vi "1_1_2.vi"() -> ()   [LabVIEW 2023, in "2025.lvlib"]
uses:
  2025.lvlib
panel:
  out "counter":i32
  out "Gauge":i32(knob)=16 scale=0.0..99.0
  out "Numeric 3":i32
  out "index of element":i32
  out "min index(es)":i32
  out "min value":i32
  out "max index(es)":i32
  out "max value":i32
  out "String":string
  out "iteration":i32
  out "Numeric 2":i32
  out "RIGHT = ON":bool
  out "x+y":i32
  out "x-y*floor(x/y)":i32
  out "floor(x/y)":i32
  out "Numeric":i32
  in  "s":bool
  out "size(s)":i32
  out "Array":i32[](array[numeric])
  # "2666 too low"
  # "6707 too high"
  # "6248 too low"
  # "6266 not it"
  # "6706 TOO HIGH"
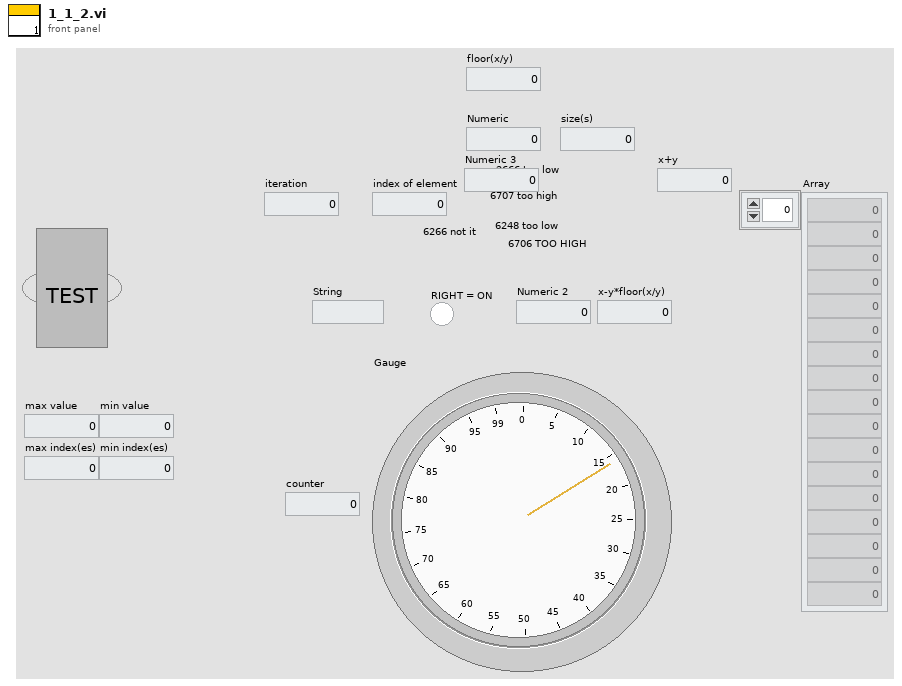
[diagram p1: front panel]
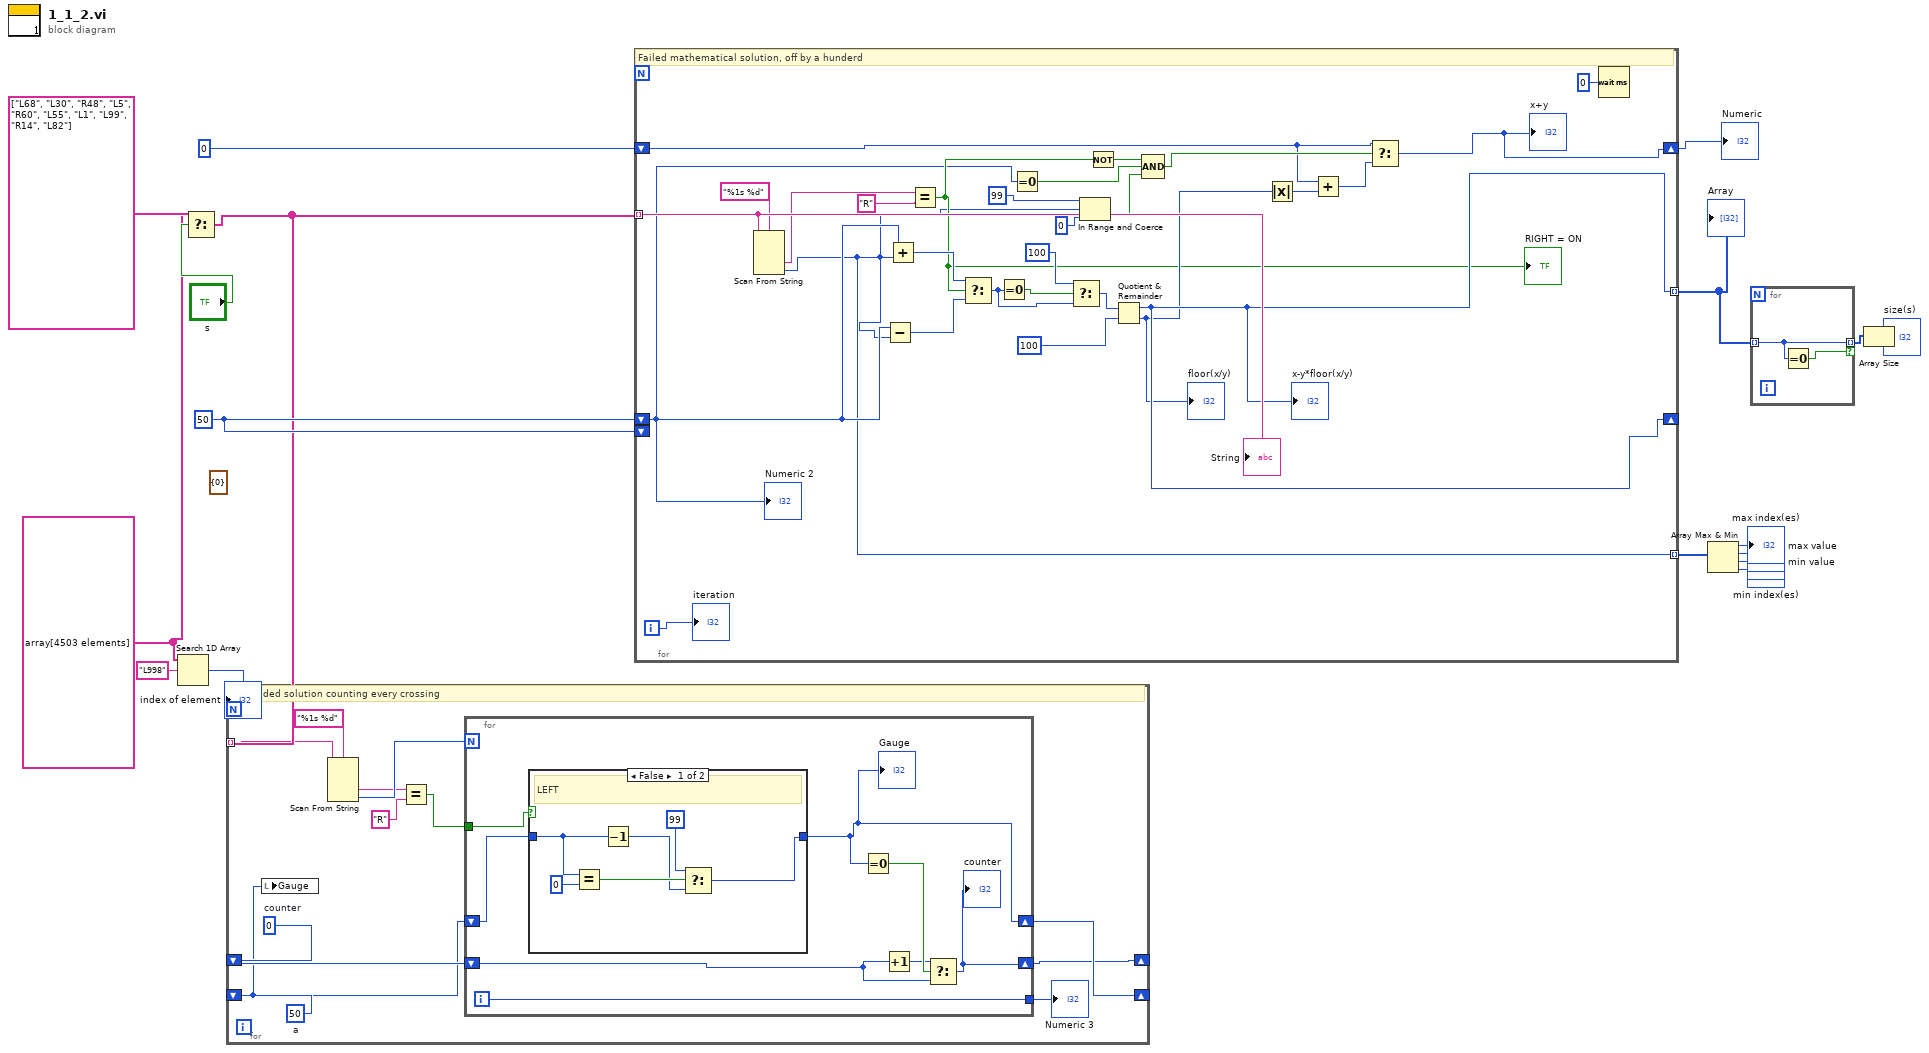
[diagram p0: block diagram]
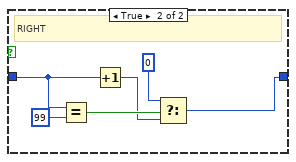
[diagram p2: hidden frame]
diagram:
  w1 = 0  # counter
  w2 = 50  # a
  (unwired) cluster{"b":i32} {"b"=0} ("Gauge")
  w6 = string[] array[4503 elements]
  w12 = 50
  n1 = Search 1D Array(1D array=w6, element="L998") -> (index of element=→"index of element":i32)  [unwired: 1 in]
  n2 = Select(t=w6, s="s", f=string[] ["L68", "L30", "R48", "L5", "R60", "L55", "L1", "L99", "R14", "L82"]) -> (s? t:f=w3:string[])
  n3 = for {
    tunnel: w3 -> [w29] mode=indexing
    shift-right: [w23] -> _
    shift-left: w2 -> [w20]
    shift-right: [w21] -> _
    shift-left: w1 -> [w22]
    # "hardcoded solution counting every crossing"
    n4 = local write "Gauge"(w20) -> ()
    n5 = Scan From String(format string="%1s %d", input string=w29) -> (output 1=w26:string, output 2=w28:i32)  [unwired: 4 in, 3 out]
    n6 = Equal?(x=w26, y="R") -> (x = y?=w25:bool)
    n7 = for {
      N: w28 -> [_]
      tunnel: [w38] -> w27
      tunnel: w25 -> [w37]
      shift-right: [w31] -> w23
      shift-left: w20 -> [w36]
      shift-right: [w35] -> w21
      shift-left: w22 -> [w33]
      i -> [w38]
      n8 = case shown="False" w37 {
        tunnel: w36 -> [w44 w50]
        tunnel: [w40 w46] -> w31
        frame False {
          # "LEFT"
          n9 = Equal?(x=w44, y=0) -> (x = y?=w42:bool)
          n10 = Decrement(x=w44) -> (x-1=w41:i32)
          n11 = Select(t=99, s=w42, f=w41) -> (s? t:f=w40:i32)
        }
        frame True {
          # "RIGHT"
          n12 = Equal?(x=w50, y=99) -> (x = y?=w48:bool)
          n13 = Increment(x=w50) -> (x+1=w47:i32)
          n14 = Select(t=0 ("y"), s=w48, f=w47) -> (s? t:f=w46:i32)
        }
      }
      "Gauge" <- w31
      n15 = Equal To 0?(x=w31) -> (x = 0?=w34:bool)
      n16 = Increment(x=w33) -> (x+1=w32:i32)
      n17 = Select(t=w32, s=w34, f=w33) -> (s? t:f=w35:i32)
      "counter" <- w35
    }
    "Numeric 3" <- w27
  }
  n18 = for {
    tunnel: w3 -> [w78] mode=indexing
    shift-right: [w68] -> _
    shift-left: w12 -> [w60]
    tunnel: [w68] -> w13 mode=indexing
    shift-right: [w52] -> w14
    shift-left: 0 -> [w54]
    shift-left: w12 -> [_]
    tunnel: [w51] -> w11 mode=indexing
    i -> [w69]
    # "Failed mathematical solution, off by a hunderd"
    n19 = Scan From String(format string="%1s %d", input string=w78) -> (output 1=w76:string, output 2=w51:i32)  [unwired: 4 in, 3 out]
    n20 = Subtract(x=w60, y=w51) -> (x-y=w73:i32)
    n21 = Add(x=w60, y=w51) -> (x+y=w74:i32)
    n22 = Equal?(x=w76, y="R") -> (x = y?=w62:bool)
    "RIGHT = ON" <- w62
    n23 = Select(t=w74, s=w62, f=w73) -> (s? t:f=w63:i32)
    n24 = Equal To 0?(x=w63) -> (x = 0?=w66:bool)
    n25 = Equal To 0?(x=w60) -> (x = 0?=w59:bool)
    n26 = Select(t=100 ("y"), s=w66, f=w63) -> (s? t:f=w65:i32)
    n27 = In Range and Coerce(upper limit=99 ("y"), x=w51, lower limit=0 ("y")) -> (In Range?=w56:bool)  [unwired: 1 out]
    n28 = Not(x=w62) -> (.not. x?=w61:bool)
    n29 = Quotient & Remainder(x=w65, y=100) -> (x-y*floor(x/y)=w68:i32, floor(x/y)=w67:i32)
    "floor(x/y)" <- w67
    "x-y*floor(x/y)" <- w68
    n30 = Compound Arithmetic op=AND(w61, w59, w56) -> (w55:bool)
    n31 = Absolute Value(x=w67) -> (abs(x)=w71:i32)
    n32 = Add(x=w54, y=w71) -> (x+y=w53:i32)
    n33 = Select(t=w54, s=w55, f=w53) -> (s? t:f=w52:i32)
    "x+y" <- w52
    n34 = Wait (ms)(milliseconds to wait=u32 0) -> ()  [unwired: 1 out]
    "Numeric 2" <- w60
    "iteration" <- w69
    "String" <- w78
  }
  "Array" <- w13
  "Numeric" <- w14
  n35 = Array Max & Min(array=w11) -> (max value=→"max value":i32, max index (indices)=→"max index(es)":i32, min value=→"min value":i32, min index (indices)=→"min index(es)":i32)
  n36 = for {
    tunnel: w13 -> [w80] mode=indexing
    tunnel: [w80] -> w18 mode=indexing if=w79
    n37 = Equal To 0?(x=w80) -> (x = 0?=w79:bool)
  }
  n38 = Array Size(array=w18) -> (size(s)=→"size(s)":i32)
